vi "stack_rotate.vi"(8 "error in (no error)":errorcluster, 9 "n":i32, 10 "index":i32, 11 "Lua in":refnum<class "Lua.lvclass">) -> (0 "error out":errorcluster, 3 "Lua out":refnum<class "Lua.lvclass">)   [LabVIEW 2020, in "Lua for LabVIEW.lvlib" / "Lua.lvclass"]
doc: "Rotates the stack elements between the valid index idx and the top of the stack. The elements are rotated n positions in the direction of the top, for a positive n, or -n positions in the direction of the bottom, for a negative n. The absolute value of n must not be greater than the size of the slice being rotated. This function cannot be called with a pseudo-index, because a pseudo-index is not an actual stack position."
uses:
  Lua.lvclass
  Lua.lvclass/Lua.ctl
  lib/lua.dll/lua.dll.lvlib
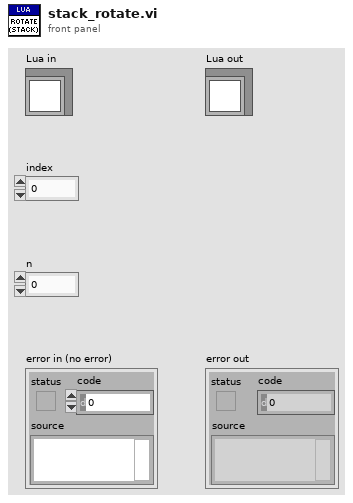
[diagram p1: front panel]
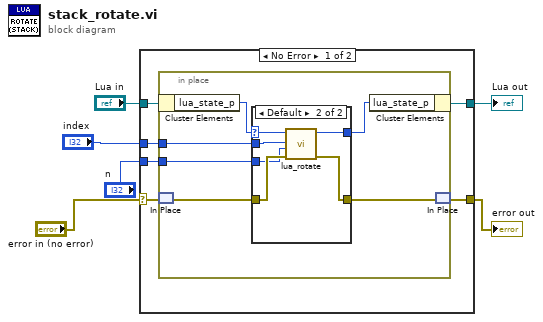
[diagram p0: block diagram]
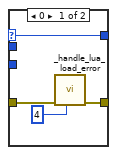
[diagram p2: hidden frame]
diagram:
  n1 = case shown="No Error" "error in (no error)" {
    selector: "error in (no error)" -> [w9 w30]
    tunnel: [w10 w30] -> w5
    tunnel: [w11 w29] -> w3
    tunnel: "Lua in" -> [w12 w29]
    tunnel: "index" -> [w8 _]
    tunnel: "n" -> [w7 _]
    frame No Error {
      n2 = in-place {
        in-place-border: w8 -> [w14]
        in-place-border: w7 -> [w13]
        n3 = in-place-cluster #1(w12) -> ("lua_state_p"=w17:u64)
        n4 = in-place-match #2(w9) -> (w16:errorcluster)
        n5 = case shown="Default" w17 {
          selector: w17 -> [w22 w27]
          tunnel: [w22 w28] -> w18
          tunnel: w16 -> [w19 w26]
          tunnel: [w20 w25] -> w15
          tunnel: w14 -> [_ w24]
          tunnel: w13 -> [_ w23]
          frame 0 {
            n6 = call "_handle_lua_load_error.vi"("lua_load errcode"=4, "error in (no error)"=w19) -> ("error out"=w20:errorcluster)  [unwired: 9 in]
          }
          frame Default {
            n7 = call "lua_rotate.vi"("error in (no error)"=w26, "n"=w23, "index"=w24, "lua_state_p"=w27) -> ("error out"=w25:errorcluster, "lua_state_p out"=w28:u64)  [unwired: 6 in]
          }
        }
        n8 = in-place-cluster #1("lua_state_p"=w18) -> (w11:refnum<class "Lua.lvclass">)
        n9 = in-place-match #2(w15) -> (w10:errorcluster)
      }
    }
    frame Error {
    }
  }
  "error out" <- w5
  "Lua out" <- w3
